vi "DSF.Engine.Timing.Get Priority.vi"(8 "error in (no error)":errorcluster, 11 "Timing in":refnum<class "DSF.Engine.Timing.lvclass">) -> (0 "error out":errorcluster, 2 "Priority":T1, 3 "Timing out":refnum<class "DSF.Engine.Timing.lvclass">)   [LabVIEW 2016, in "DSF.Engine.lvlib" / "DSF.Engine.Timing.lvclass"]
uses:
  DSF.Engine.Timing.lvclass
  Shared/Typedefs/DSF.Shared.Typedefs.Scalars.Priority.ctl
  DSF.Engine.Timing.lvclass/DSF.Engine.Timing.ctl
  DSF.Shared.lvlib
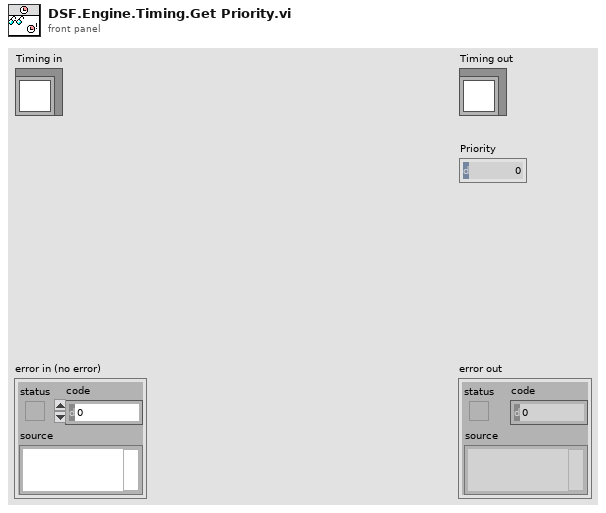
[diagram p1: front panel]
types:
  T1 = typedef "DSF.Shared.lvlib/DSF.Shared.Typedefs.Scalars.Priority.ctl" = u64
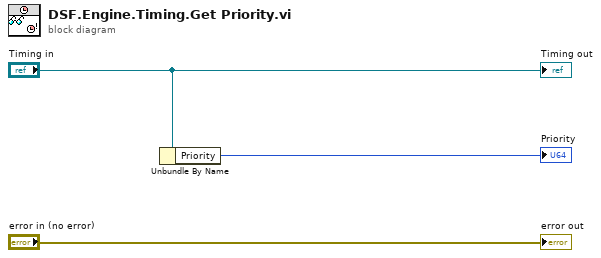
[diagram p0: block diagram]
diagram:
  n1 = Unbundle By Name("Timing in") -> ("Priority"=→"Priority":T1)
  "error out" <- "error in (no error)"
  "Timing out" <- "Timing in"
